vi "界面UI.vi"() -> ()   [LabVIEW 2016, in "超标留样.lvlib"]
panel:
  out "超标留样运行状态":T1(xcontrol)
  in  "外控留样设置":bool
  in  "外控留样读取":bool
  in  "串口重开":bool
  in  "读取选择":string(combo)
  in  "超标留样设置":bool
  in  "超标留样读取":bool
  in  "VISA resource name":refnum<visa-resource-name>="COM2" caption="VISA资源名称"
  in  "写入缓冲区":string
  in  "采样模式":enum16{"定时留样", "时间等比", "同步留样", "外控留样", "超标留样"}(ring)
  in  "采样启动":bool
  in  "切换停止":bool
  in  "切换运行":bool
  in  "时间校准":bool
  out "仪器状态":T1 {"仪器时间" format="%<%Y/%m/%d %H:%M:%S>T"; "门状态" items=["关闭", "打开"]; "采样模式" items=["定时留样"=1, "时间等比"=2, "同步留样"=3, "外控留样"=4, "超标留样"=5]; "工作进程" items=["停止中"=0, "启动延时"=1, "外置泵延时"=2, "管路润洗"=3, "管存"=4, "留样"=5, "出水管路排空"=6, "采水管路排空"=7, "待机"=13]; "工作状态" items=["停止", "运行", "系统初始化"]}
  out "读取缓冲区":string
  out "source":string
  out "通讯":bool
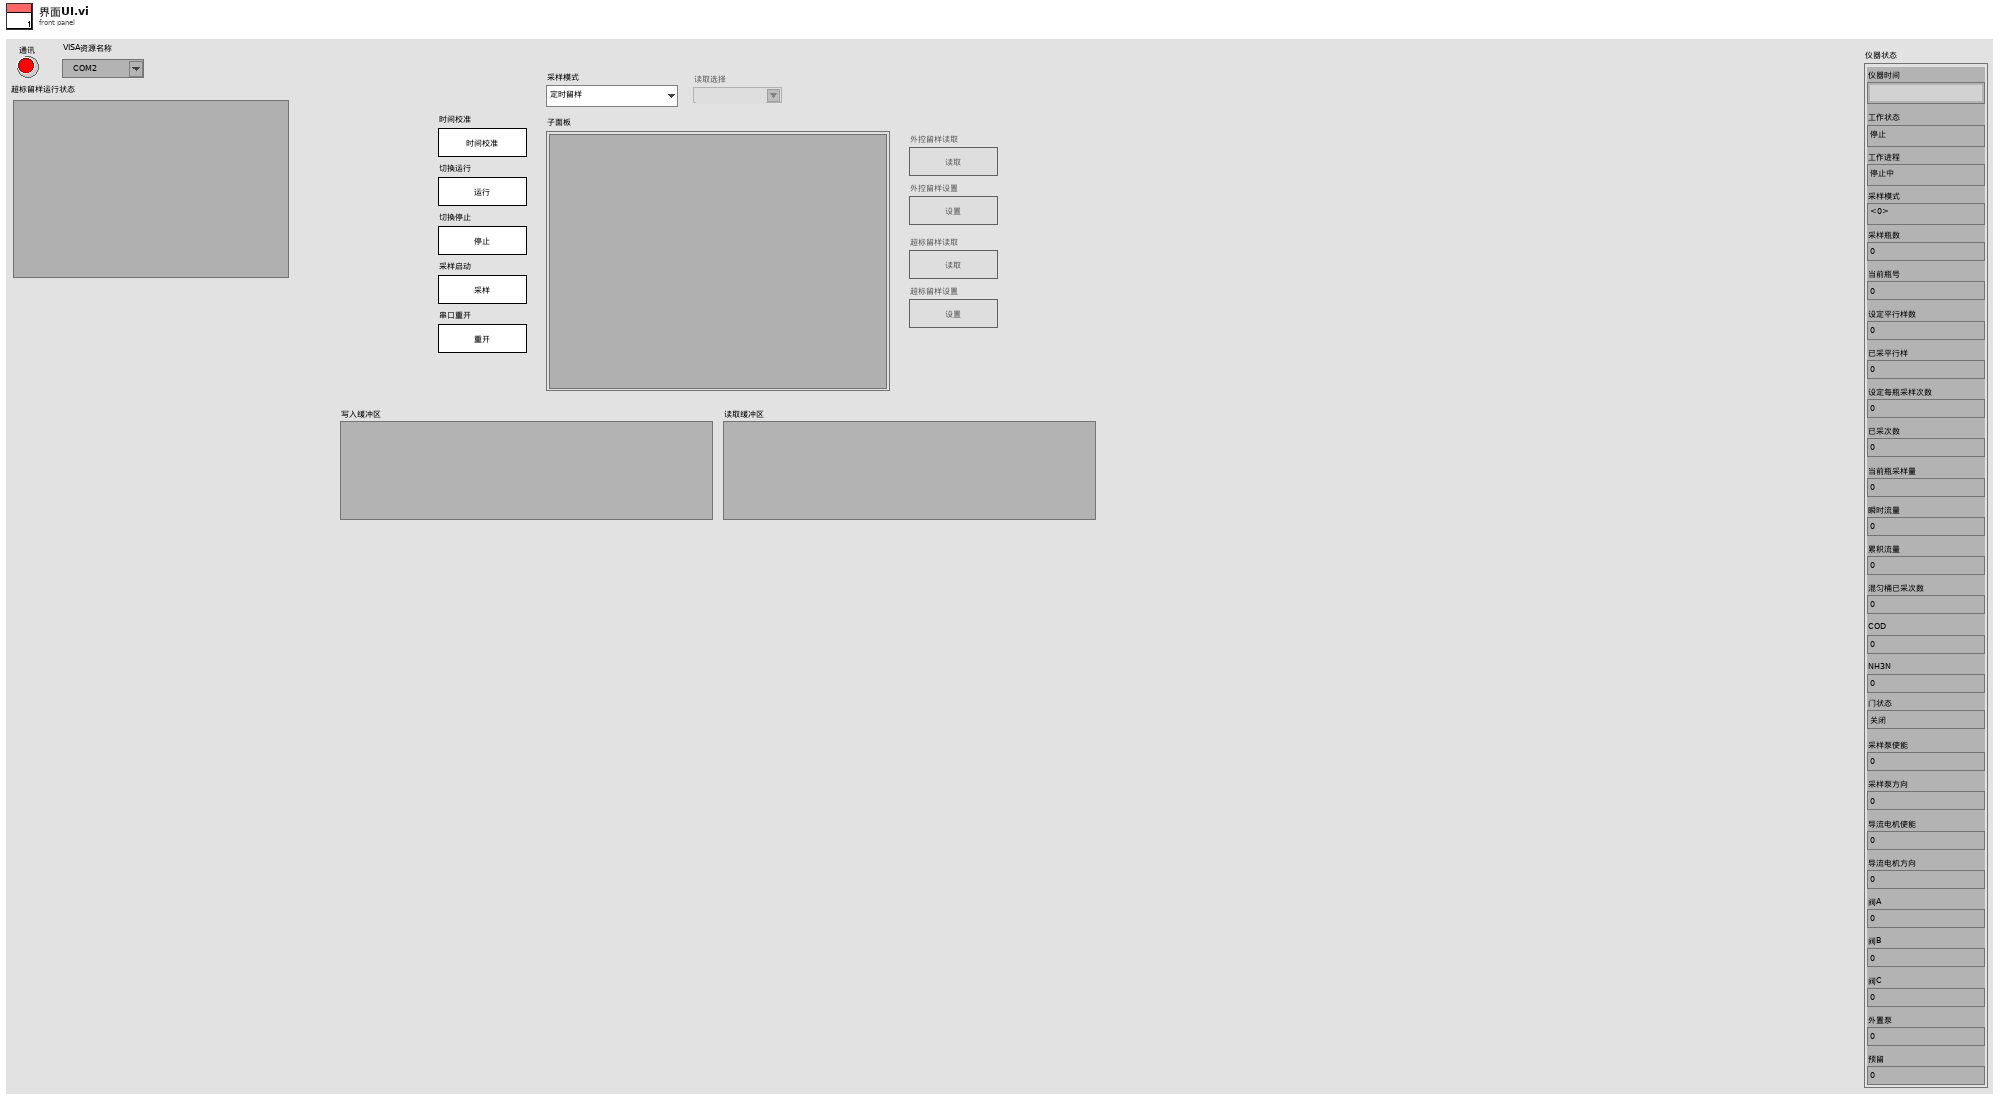
[diagram p1: front panel]
types:
  T1 = cluster{"仪器时间":timestamp, "工作状态":u16, "工作进程":u16, "采样模式":u16, "采样瓶数":dbl, "当前瓶号":dbl, "设定平行样数":dbl, "已采平行样":dbl, "设定每瓶采样次数":dbl, "已采次数":dbl, "当前瓶采样量":dbl, "瞬时流量":dbl, "累积流量":dbl, "混匀桶已采次数":dbl, "COD":dbl, "NH3N":dbl, "门状态":u16, "采样泵使能":dbl, "采样泵方向":dbl, "导流电机使能":dbl, "导流电机方向":dbl, "阀A":dbl, "阀B":dbl, "阀C":dbl, "外置泵":dbl, "预留":dbl}
  T2 = enum32{"Bad", "Idle", "Run top level", "Running"}
  T3 = cluster{"当前瓶号：":dbl, "平行样：":dbl, "留样瓶数：":dbl, "每瓶次数：":dbl, "每次留样：":dbl}
  T4 = cluster{"当前瓶号：":dbl, "平行样：":dbl, "留样瓶数：":dbl, "每瓶次数：":dbl, "每次留样：":dbl, "时间间隔：":dbl, "COD联机：":u16, "氨氮联机：":u16, "4mA浓度：":dbl, "20mA浓度：":dbl, "超标浓度：":dbl, "4mA浓度：":dbl, "20mA浓度:":dbl, "超标浓度：":dbl}
  T5 = enum8{"Enabled", "Disabled", "Disabled and Grayed Out"}
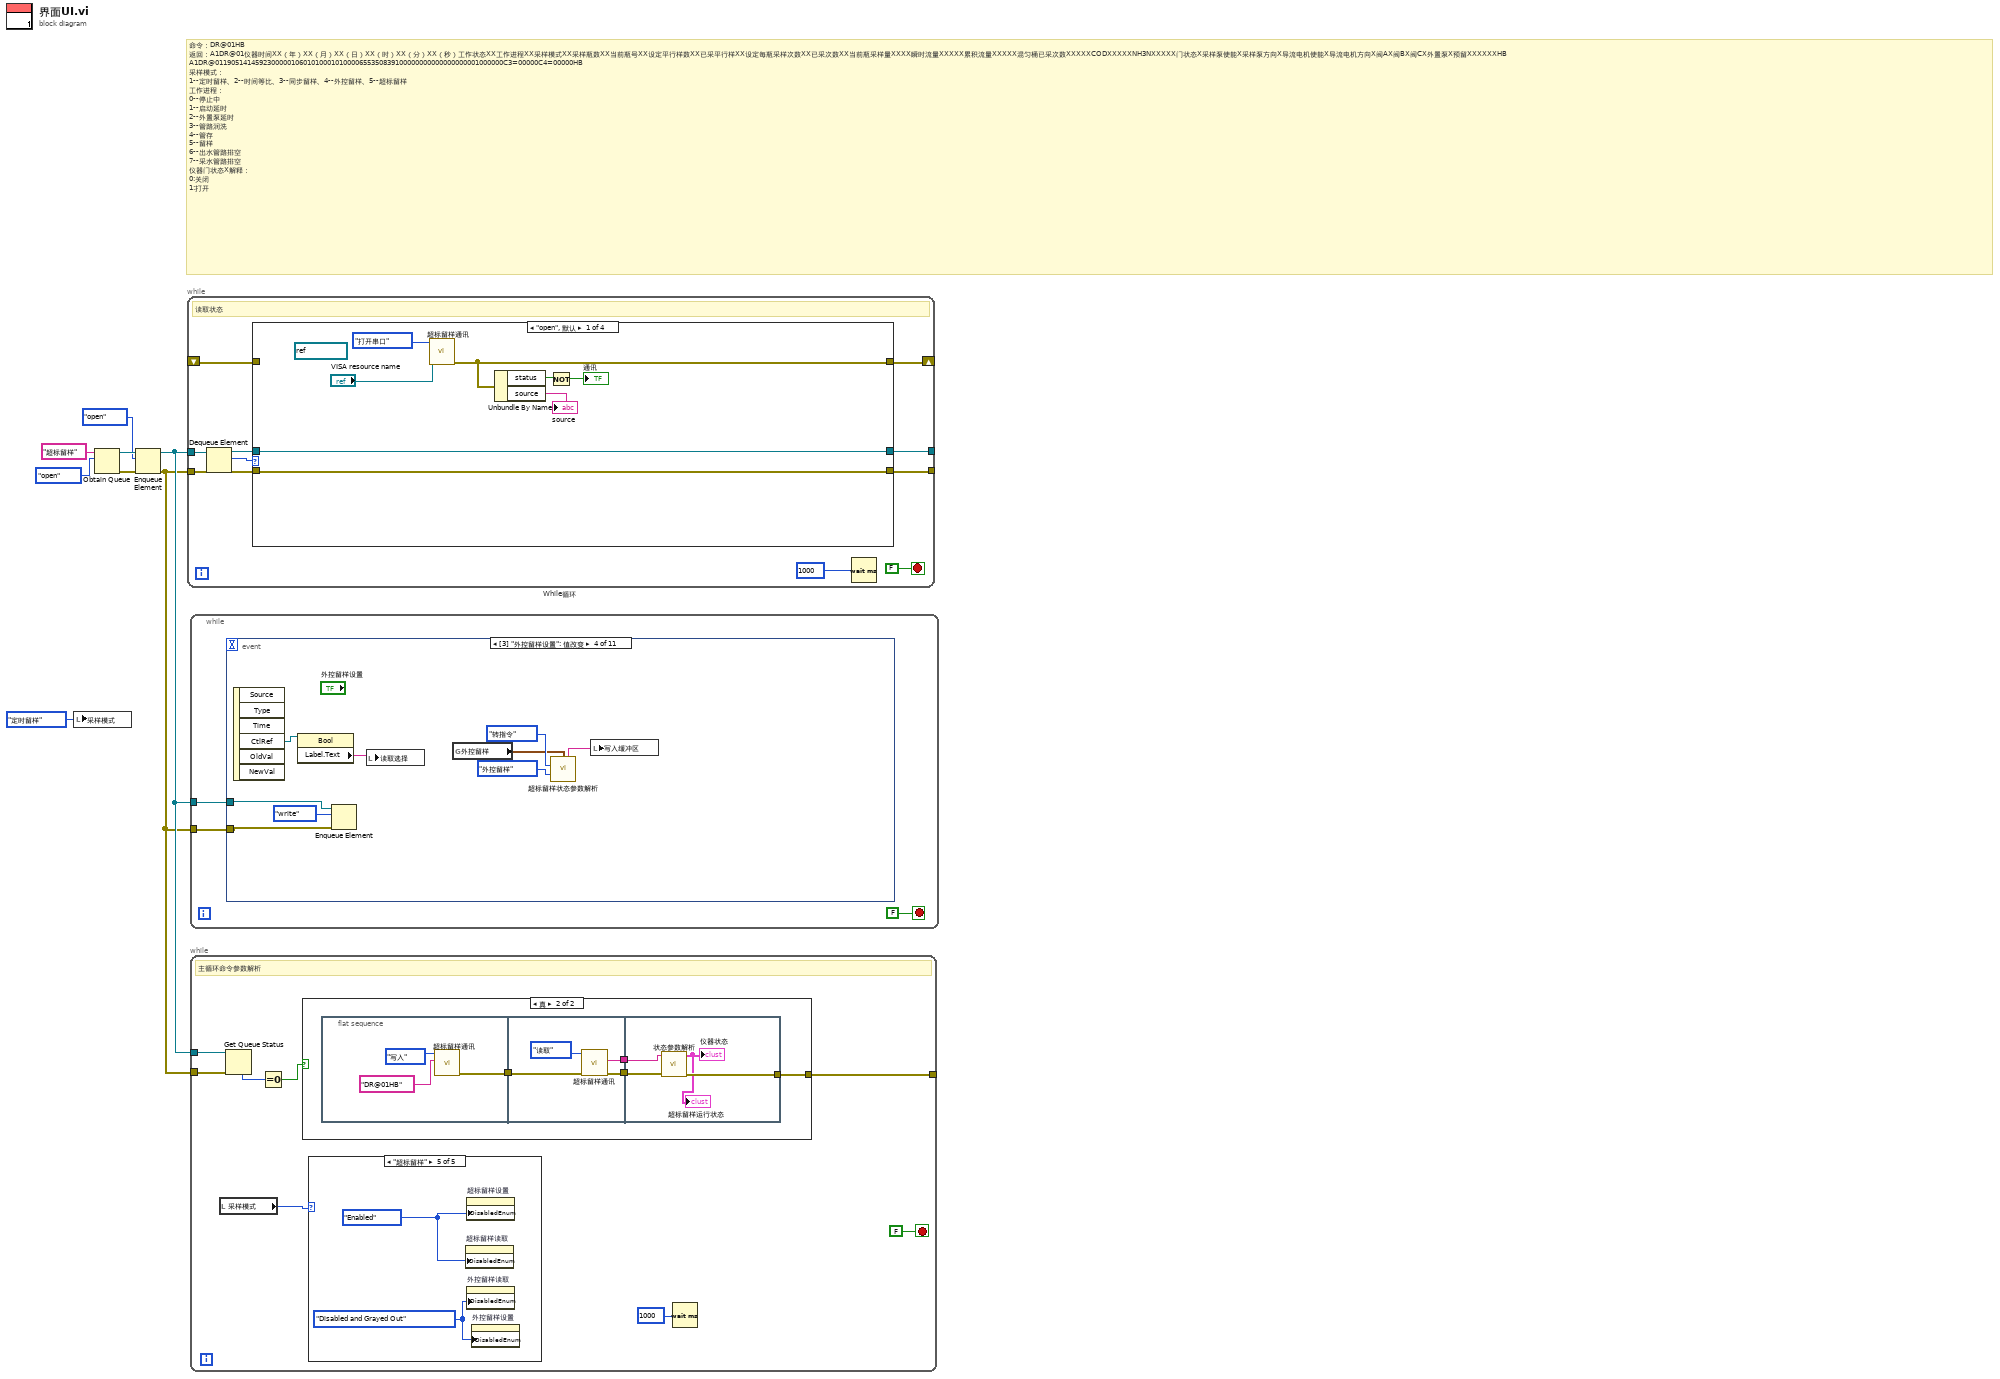
[diagram p0: block diagram]
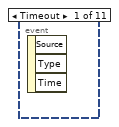
[diagram p2: hidden frame]
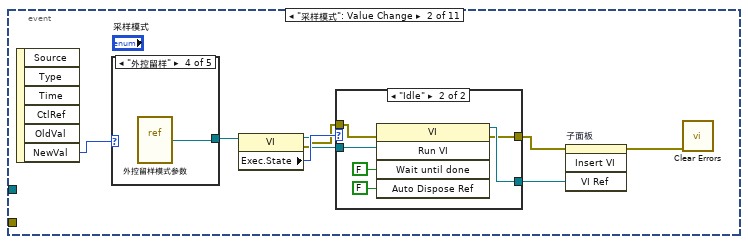
[diagram p3: hidden frame]
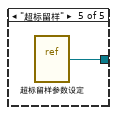
[diagram p8: hidden frame]
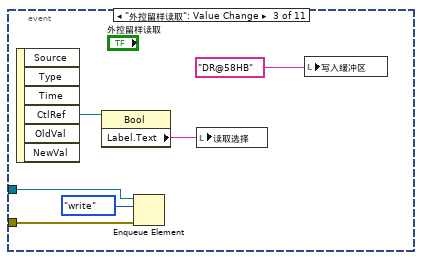
[diagram p9: hidden frame]
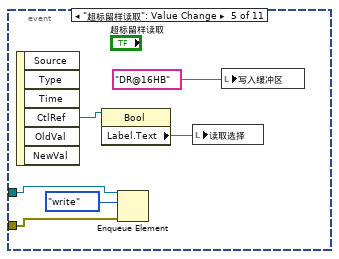
[diagram p10: hidden frame]
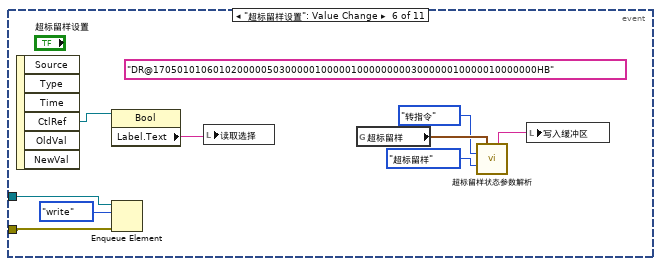
[diagram p11: hidden frame]
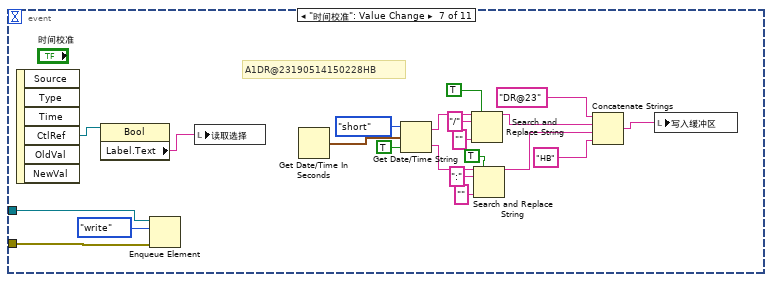
[diagram p12: hidden frame]
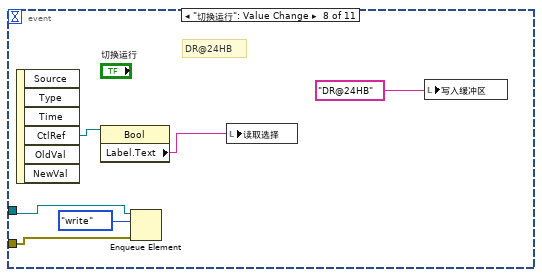
[diagram p13: hidden frame]
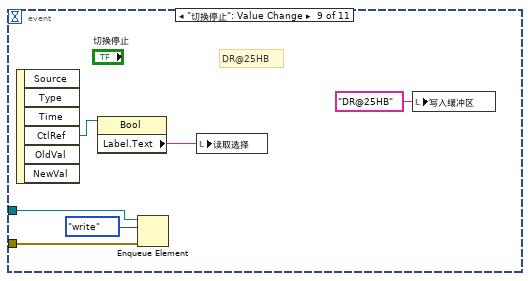
[diagram p14: hidden frame]
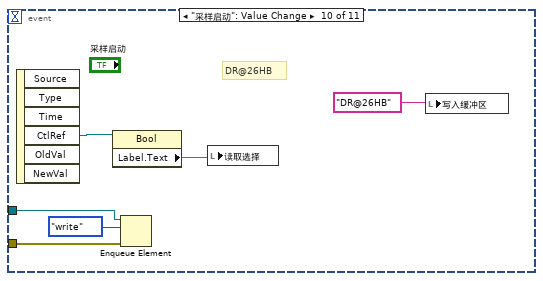
[diagram p15: hidden frame]
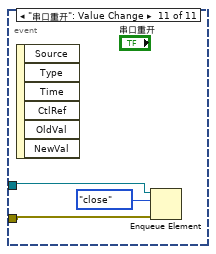
[diagram p16: hidden frame]
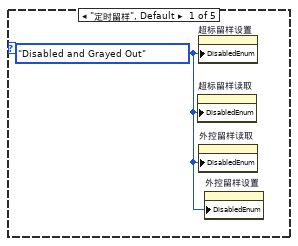
[diagram p18: hidden frame]
diagram:
  # "命令：DR@01HB\n返回：A1DR@01仪器时间XX（年）XX（月）XX（日）XX（时）XX（分）XX（秒）工作状态XX工作进程XX采样模式XX采样瓶数XX当前瓶号XX设定平行样数XX已采平行样XX设定每瓶采样次数XX已采次数XX当前瓶采样量XXXX瞬时流量XXXXX累积流量XXXXX混匀桶已采次数XXXXXCODXXXXXNH3NXXXXX门状态X采样泵使能X采样泵方向X导流电机使能X导流电机方向X阀AX阀BX阀CX外置泵X预留XXXXXXHB\nA1DR@011905141459230000010601010001010000655350839100000000000000000001000000C3=00000C4=00000HB\n采样模式：\n1--定时留样、2--时间等比、3--同步留样、4--外控留样、5--超标留样\n工作进程：\n0--停止中\n1--启动延时\n2--外置泵延时\n3--管路润洗\n4--管存\n5--留样\n6--出水管路排空\n7--采水管路排空\n仪器门状态X解释：\n0:关闭\n1:打开"
  n1 = local write "采样模式"(enum16{"定时留样", "时间等比", "同步留样", "外控留样", "超标留样"}."定时留样" ("采样模式")) -> ()
  n2 = Obtain Queue(name (unnamed)="超标留样" ("名称（未命名）"), element data type=enum16{"open", "read", "write", "close"}."open") -> (queue out=w6:refnum<queue>, error out=w5:errorcluster)  [unwired: 3 in, 1 out]
  n3 = Enqueue Element(queue=w6, element=enum16{"open", "read", "write", "close"}."open", error in (no error)=w5) -> (queue out=w2:refnum<queue>, error out=w1:errorcluster)  [unwired: 1 in, 1 out]
  n4 = while "While循环" {
    tunnel: w2 -> [w17]
    tunnel: w1 -> [w16]
    tunnel: [w12] -> _
    tunnel: [w11] -> _
    shift-right: [w10] -> _
    shift-left: _ -> [w9]
    stop <- FALSE stop-if-true
    # "读取状态"
    n5 = Dequeue Element(queue=w17, error in (no error)=w16) -> (queue out=w14:refnum<queue>, element=w15:enum16{"open", "read", "write", "close"}, error out=w13:errorcluster)  [unwired: 1 in, 1 out]
    n6 = case shown="\"open\", 默认" w15 {
      tunnel: [w26 w33 w56 w68] -> w10
      tunnel: w14 -> [w21 w31 w61 w67]
      tunnel: w13 -> [w20 w30 w60 w66]
      tunnel: [w21 w31 w59 w64] -> w12
      tunnel: [w20 w30 w58 w63] -> w11
      tunnel: w9 -> [_ w34 w57 w70]
      frame "open", Default {
        (unwired) refnum<visa-resource-name> "COM2" ("VISA resource name")
        n7 = call "超标留样通讯.vi"("VISA resource name"="VISA resource name", "功能输入"=enum16{"打开串口", "写入", "读取", "关闭串口"}."打开串口") -> ("error out"=w26:errorcluster)  [unwired: 7 in, 2 out]
        n8 = Unbundle By Name(w26) -> ("status"=w25:bool, "source"=→"source":string)
        n9 = Not(x=w25) -> (.not. x?=→"通讯":bool)
      }
      frame "read" {
        n10 = call "超标留样通讯.vi"("error in (no error)"=w34, "功能输入"=enum16{"打开串口", "写入", "读取", "关闭串口"}."读取") -> ("error out"=w33:errorcluster, "读取缓冲区"=w28:string)  [unwired: 7 in, 1 out]
        "读取缓冲区" <- w28
        n11 = case shown="\"外控留样读取\"" "读取选择" {
          tunnel: w28 -> [w35 w42 w53]
          frame "超标留样读取" {
            n12 = flat-sequence {
              tunnel: w35 -> [w38]
              frame #0 {
                n13 = call "超标留样状态参数解析.vi"("输入字符串"=w38, "解析/转指令"=enum16{"解析", "转指令"}."解析", "模式选择"=enum16{"外控留样", "超标留样"}."超标留样") -> ()  [unwired: 11 in, 2 out]
              }
              frame #1 {
                n14 = global write "超标留样全局.vi" "读取更新"(TRUE ("读取更新")) -> ()
              }
              frame #2 {
                n15 = Wait (ms)(milliseconds to wait=u32 500 ("等待时间（毫秒）")) -> ()  [unwired: 1 out]
              }
              frame #3 {
                n16 = global write "超标留样全局.vi" "读取更新"(FALSE ("读取更新")) -> ()
              }
            }
          }
          frame "外控留样读取" {
            n17 = flat-sequence {
              tunnel: w42 -> [w43]
              frame #0 {
                n18 = call "超标留样状态参数解析.vi"("输入字符串"=w43, "解析/转指令"=enum16{"解析", "转指令"}."解析", "模式选择"=enum16{"外控留样", "超标留样"}."外控留样") -> ()  [unwired: 11 in, 2 out]
              }
              frame #1 {
                n19 = global write "超标留样全局.vi" "外控留样读取更新"(TRUE ("读取更新")) -> ()
              }
              frame #2 {
                n20 = Wait (ms)(milliseconds to wait=u32 500 ("等待时间（毫秒）")) -> ()  [unwired: 1 out]
              }
              frame #3 {
                n21 = global write "超标留样全局.vi" "外控留样读取更新"(FALSE ("读取更新")) -> ()
              }
            }
          }
          frame "超标留样设置", Default {
            n22 = String Subset(string=w53, offset (0)=5 ("偏移量(0)")) -> (substring=w51:string)  [unwired: 1 in]
            n23 = Search/Split String(string=w51, search string/char (-)="HB" ("搜索字符串/字符(-)")) -> (substring before match=w49:string)  [unwired: 1 in, 2 out]
            n24 = One Button Dialog(message=w49) -> ()  [unwired: 1 in, 1 out]
          }
        }
      }
      frame "write" {
        n25 = call "超标留样通讯.vi"("error in (no error)"=w57, "写入缓冲区"="写入缓冲区", "功能输入"=enum16{"打开串口", "写入", "读取", "关闭串口"}."写入") -> ("error out"=w56:errorcluster)  [unwired: 6 in, 2 out]
        n26 = Enqueue Element(queue=w61, element=enum16{"open", "read", "write", "close"}."read" ("元素"), error in (no error)=w60) -> (queue out=w59:refnum<queue>, error out=w58:errorcluster)  [unwired: 1 in, 1 out]
      }
      frame "close" {
        n27 = call "超标留样通讯.vi"("error in (no error)"=w70, "功能输入"=enum16{"打开串口", "写入", "读取", "关闭串口"}."关闭串口") -> ("error out"=w68:errorcluster)  [unwired: 7 in, 2 out]
        n28 = Enqueue Element(queue=w67, element=enum16{"open", "read", "write", "close"}."open" ("元素"), error in (no error)=w66) -> (queue out=w64:refnum<queue>, error out=w63:errorcluster)  [unwired: 1 in, 1 out]
      }
    }
    n29 = Wait (ms)(milliseconds to wait=u32 1000 ("等待时间（毫秒）")) -> ()  [unwired: 1 out]
  }
  n30 = while {
    tunnel: w2 -> [w72]
    tunnel: w1 -> [w71]
    stop <- FALSE stop-if-true
    n31 = event shown="[3] \"外控留样设置\": 值改变" {
      selector: _ -> [_ _ _ _ _ _ _ _ _ _ _]
      dyn-events: _ -> [_ _ _ _ _ _ _ _ _ _ _]
      timeout: _ -> [_ _ _ _ _ _ _ _ _ _ _]
      tunnel: w72 -> [_ _ w94 w105 w110 w120 w141 w146 w152 w158 w162]
      tunnel: w71 -> [_ _ w95 w104 w109 w119 w140 w145 w151 w157 w161]
      event Timeout {
        n32 = event-data() -> ()  [unwired: 1 in, 3 out]
      }
      event "采样模式": Value Change {
        n33 = event-data() -> ("NewVal"=w81:enum16{"定时留样", "时间等比", "同步留样", "外控留样", "超标留样"})  [unwired: 1 in, 5 out]
        n34 = case shown="\"外控留样\"" w81 {
          tunnel: [_ _ _ w90 w91] -> w80
          frame "定时留样", Default {
          }
          frame "时间等比" {
          }
          frame "同步留样" {
          }
          frame "外控留样" {
            n35 = vi-ref "外控留样模式参数.vi"() -> (w90:refnum<vi>)
          }
          frame "超标留样" {
            n36 = vi-ref "超标留样参数设定.vi"() -> (w91:refnum<vi>)
          }
        }
        n37 = property class="VI"(reference=w80) -> (reference out=w78:refnum<vi>, error out=w76:errorcluster, "Exec.State"=w79:T2)  [unwired: 1 in]
        n38 = case shown="\"Idle\"" w79 {
          tunnel: w78 -> [w83 w89]
          tunnel: [w83 w86] -> w77
          tunnel: w76 -> [w82 w85]
          tunnel: [w82 w84] -> w75
          frame "Bad", Default {
          }
          frame "Idle" {
            n39 = invoke class="VI" method="Run VI"(reference=w89, error in=w85, "Wait until done"=FALSE ("结束前等待"), "Auto Dispose Ref"=FALSE ("自动销毁引用")) -> (reference out=w86:refnum<vi>, error out=w84:errorcluster)  [unwired: 1 in, 3 out]
          }
        }
        n40 = invoke on="子面板" class="SubPnl" method="Insert VI"(error in=w75, "VI Ref"=w77) -> (error out=w74:errorcluster)  [unwired: 2 in, 3 out]
        n41 = call <vilib>:"Clear Errors.vi"("error in (no error)"=w74) -> ()  [unwired: 5 in, 2 out]
      }
      event "外控留样读取": Value Change {
        n42 = event-data() -> ("CtlRef"=w93:refnum<vi>)  [unwired: 1 in, 5 out]
        n43 = property class="Bool"(reference=w93) -> ("Label.Text"=w92:string)  [unwired: 1 in, 2 out]
        n44 = Enqueue Element(queue=w94, element=enum16{"open", "read", "write", "close"}."write" ("元素"), error in (no error)=w95) -> ()  [unwired: 1 in, 3 out]
        n45 = local write "读取选择"(w92) -> ()
        n46 = local write "写入缓冲区"("DR@58HB") -> ()
      }
      event "外控留样设置": Value Change {
        n47 = event-data() -> ("CtlRef"=w99:refnum<vi>)  [unwired: 1 in, 5 out]
        n48 = property class="Bool"(reference=w99) -> ("Label.Text"=w98:string)  [unwired: 1 in, 2 out]
        n49 = Enqueue Element(queue=w105, element=enum16{"open", "read", "write", "close"}."write" ("元素"), error in (no error)=w104) -> ()  [unwired: 1 in, 3 out]
        n50 = local write "读取选择"(w98) -> ()
        n51 = global read "超标留样全局.vi" "外控留样"() -> (w100:T3)
        n52 = call "超标留样状态参数解析.vi"("外控留样"=w100, "解析/转指令"=enum16{"解析", "转指令"}."转指令", "模式选择"=enum16{"外控留样", "超标留样"}."外控留样") -> ("输出字符串"=w101:string)  [unwired: 11 in, 1 out]
        n53 = local write "写入缓冲区"(w101) -> ()
      }
      event "超标留样读取": Value Change {
        n54 = event-data() -> ("CtlRef"=w108:refnum<vi>)  [unwired: 1 in, 5 out]
        n55 = property class="Bool"(reference=w108) -> ("Label.Text"=w107:string)  [unwired: 1 in, 2 out]
        n56 = Enqueue Element(queue=w110, element=enum16{"open", "read", "write", "close"}."write" ("元素"), error in (no error)=w109) -> ()  [unwired: 1 in, 3 out]
        n57 = local write "读取选择"(w107) -> ()
        n58 = local write "写入缓冲区"("DR@16HB") -> ()
      }
      event "超标留样设置": Value Change {
        (unwired) "DR@1705010106010200000503000001000001000000000300000010000010000000HB"
        n59 = event-data() -> ("CtlRef"=w114:refnum<vi>)  [unwired: 1 in, 5 out]
        n60 = property class="Bool"(reference=w114) -> ("Label.Text"=w113:string)  [unwired: 1 in, 2 out]
        n61 = Enqueue Element(queue=w120, element=enum16{"open", "read", "write", "close"}."write" ("元素"), error in (no error)=w119) -> ()  [unwired: 1 in, 3 out]
        n62 = local write "读取选择"(w113) -> ()
        n63 = global read "超标留样全局.vi" "超标留样"() -> (w118:T4)
        n64 = call "超标留样状态参数解析.vi"("超标留样"=w118, "解析/转指令"=enum16{"解析", "转指令"}."转指令", "模式选择"=enum16{"外控留样", "超标留样"}."超标留样") -> ("输出字符串"=w115:string)  [unwired: 11 in, 1 out]
        n65 = local write "写入缓冲区"(w115) -> ()
      }
      event "时间校准": Value Change {
        # "A1DR@23190514150228HB"
        n66 = event-data() -> ("CtlRef"=w123:refnum<vi>)  [unwired: 1 in, 5 out]
        n67 = property class="Bool"(reference=w123) -> ("Label.Text"=w122:string)  [unwired: 1 in, 2 out]
        n68 = Enqueue Element(queue=w141, element=enum16{"open", "read", "write", "close"}."write" ("元素"), error in (no error)=w140) -> ()  [unwired: 1 in, 3 out]
        n69 = local write "读取选择"(w122) -> ()
        n70 = Get Date/Time In Seconds() -> (seconds since 1Jan1904=w136:timestamp)
        n71 = Get Date/Time String(date format (0)=enum16{"short", "long", "abbreviated"}."short" ("日期格式(0)"), seconds (now)=w136, want seconds? (F)=TRUE ("需要秒？(F)")) -> (date string=w135:string, time string=w128:string)
        n72 = Search and Replace String(replace all?=TRUE ("替换全部？(F)"), input string=w135, search string="/" ("搜索字符串"), replace string="" ("替换字符串(\"\")")) -> (result string=w127:string)  [unwired: 4 in, 3 out]
        n73 = Search and Replace String(replace all?=TRUE ("替换全部？(F)"), input string=w128, search string=":" ("搜索字符串"), replace string="" ("替换字符串(\"\")")) -> (result string=w126:string)  [unwired: 4 in, 3 out]
        n74 = Concatenate Strings("DR@23" ("写入缓冲区"), w127, w126, "HB" ("写入缓冲区")) -> (w124:string)
        n75 = local write "写入缓冲区"(w124) -> ()
      }
      event "切换运行": Value Change {
        # "DR@24HB"
        n76 = event-data() -> ("CtlRef"=w144:refnum<vi>)  [unwired: 1 in, 5 out]
        n77 = property class="Bool"(reference=w144) -> ("Label.Text"=w143:string)  [unwired: 1 in, 2 out]
        n78 = Enqueue Element(queue=w146, element=enum16{"open", "read", "write", "close"}."write" ("元素"), error in (no error)=w145) -> ()  [unwired: 1 in, 3 out]
        n79 = local write "读取选择"(w143) -> ()
        n80 = local write "写入缓冲区"("DR@24HB") -> ()
      }
      event "切换停止": Value Change {
        # "DR@25HB"
        n81 = event-data() -> ("CtlRef"=w150:refnum<vi>)  [unwired: 1 in, 5 out]
        n82 = property class="Bool"(reference=w150) -> ("Label.Text"=w149:string)  [unwired: 1 in, 2 out]
        n83 = Enqueue Element(queue=w152, element=enum16{"open", "read", "write", "close"}."write" ("元素"), error in (no error)=w151) -> ()  [unwired: 1 in, 3 out]
        n84 = local write "读取选择"(w149) -> ()
        n85 = local write "写入缓冲区"("DR@25HB" ("写入缓冲区")) -> ()
      }
      event "采样启动": Value Change {
        # "DR@26HB"
        n86 = event-data() -> ("CtlRef"=w156:refnum<vi>)  [unwired: 1 in, 5 out]
        n87 = property class="Bool"(reference=w156) -> ("Label.Text"=w155:string)  [unwired: 1 in, 2 out]
        n88 = Enqueue Element(queue=w158, element=enum16{"open", "read", "write", "close"}."write" ("元素"), error in (no error)=w157) -> ()  [unwired: 1 in, 3 out]
        n89 = local write "读取选择"(w155) -> ()
        n90 = local write "写入缓冲区"("DR@26HB") -> ()
      }
      event "串口重开": Value Change {
        n91 = event-data() -> ()  [unwired: 1 in, 6 out]
        n92 = Enqueue Element(queue=w162, element=enum16{"open", "read", "write", "close"}."close" ("元素"), error in (no error)=w161) -> ()  [unwired: 1 in, 3 out]
      }
    }
  }
  n93 = while {
    tunnel: [w169] -> _
    tunnel: w2 -> [w167]
    tunnel: w1 -> [w166]
    stop <- FALSE stop-if-true
    # "主循环命令参数解析"
    n94 = local read "采样模式"() -> (w168:enum16{"定时留样", "时间等比", "同步留样", "外控留样", "超标留样"})
    n95 = Get Queue Status(queue=w167, error in (no error)=w166) -> (# elements in queue=w165:i32)  [unwired: 1 in, 7 out]
    n96 = Equal To 0?(x=w165) -> (x = 0?=w164:bool)
    n97 = case shown="真" w164 {
      tunnel: [_ w172] -> w169
      frame False {
      }
      frame True {
        n98 = flat-sequence {
          tunnel: [w176] -> w175
          tunnel: w175 -> [w181]
          tunnel: [w180] -> w174
          tunnel: [w179] -> w173
          tunnel: w174 -> [w186]
          tunnel: w173 -> [w185]
          tunnel: [w184] -> w172
          frame #0 {
            n99 = call "超标留样通讯.vi"("写入缓冲区"="DR@01HB", "功能输入"=enum16{"打开串口", "写入", "读取", "关闭串口"}."写入") -> ("error out"=w176:errorcluster)  [unwired: 7 in, 2 out]
          }
          frame #1 {
            n100 = call "超标留样通讯.vi"("error in (no error)"=w181, "功能输入"=enum16{"打开串口", "写入", "读取", "关闭串口"}."读取") -> ("error out"=w180:errorcluster, "读取缓冲区"=w179:string)  [unwired: 7 in, 1 out]
          }
          frame #2 {
            n101 = call "状态参数解析.vi"("error in (no error)"=w186, "字符串"=w185) -> ("error out"=w184:errorcluster, "簇"=→"仪器状态" →"超标留样运行状态":T1)  [unwired: 8 in]
          }
        }
      }
    }
    n102 = case shown="\"超标留样\"" w168 {
      frame "定时留样", Default {
        w187 = T5."Disabled and Grayed Out" ("禁用")
        n103 = property on="超标留样读取" class="Bool"("DisabledEnum"=w187) -> ()  [unwired: 2 in, 2 out]
        n104 = property on="超标留样设置" class="Bool"("DisabledEnum"=w187) -> ()  [unwired: 2 in, 2 out]
        n105 = property on="外控留样读取" class="Bool"("DisabledEnum"=w187) -> ()  [unwired: 2 in, 2 out]
        n106 = property on="外控留样设置" class="Bool"("DisabledEnum"=w187) -> ()  [unwired: 2 in, 2 out]
      }
      frame "时间等比" {
      }
      frame "同步留样" {
      }
      frame "外控留样" {
        w188 = T5."Enabled" ("禁用")
        w189 = T5."Disabled and Grayed Out" ("禁用")
        n107 = property on="超标留样读取" class="Bool"("DisabledEnum"=w189) -> ()  [unwired: 2 in, 2 out]
        n108 = property on="超标留样设置" class="Bool"("DisabledEnum"=w189) -> ()  [unwired: 2 in, 2 out]
        n109 = property on="外控留样读取" class="Bool"("DisabledEnum"=w188) -> ()  [unwired: 2 in, 2 out]
        n110 = property on="外控留样设置" class="Bool"("DisabledEnum"=w188) -> ()  [unwired: 2 in, 2 out]
      }
      frame "超标留样" {
        w190 = T5."Enabled" ("禁用")
        w191 = T5."Disabled and Grayed Out" ("禁用")
        n111 = property on="超标留样读取" class="Bool"("DisabledEnum"=w190) -> ()  [unwired: 2 in, 2 out]
        n112 = property on="超标留样设置" class="Bool"("DisabledEnum"=w190) -> ()  [unwired: 2 in, 2 out]
        n113 = property on="外控留样读取" class="Bool"("DisabledEnum"=w191) -> ()  [unwired: 2 in, 2 out]
        n114 = property on="外控留样设置" class="Bool"("DisabledEnum"=w191) -> ()  [unwired: 2 in, 2 out]
      }
    }
    n115 = Wait (ms)(milliseconds to wait=u32 1000 ("等待时间（毫秒）")) -> ()  [unwired: 1 out]
  }
